vi "Lockin.Sample.vi"(8 "error in (no error)":errorcluster, 11 "Lockin.DAQ":refnum<class "Instrument.DAQ.lvclass">) -> (0 "error out":errorcluster, 2 "Results":T1 {"Results (Dictionary)"."value" format="%#_6p"}, 3 "Lockin.DAQ out":refnum<class "Instrument.DAQ.lvclass">)   [LabVIEW 2019, in "Instrument.Lockin.lvlib" / "Instrument.DAQ.lvclass"]
uses:
  Instrument.DAQ.lvclass
  Typedefs/Results--Cluster.ctl
  Instrument.DAQ.lvclass/Instrument.DAQ.ctl
  <vilib>/Analysis/baseanly.llb/Mean (DBL).vi
  <vilib>/Analysis/NI_AALBase.lvlib
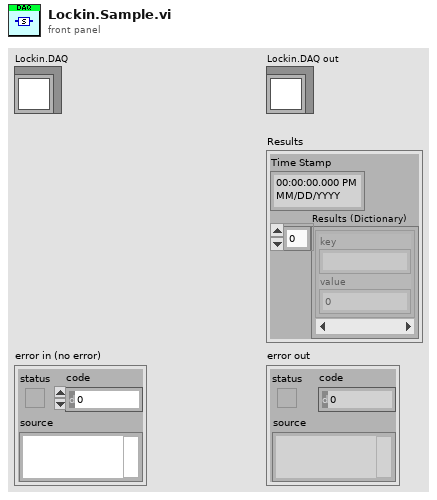
[diagram p1: front panel]
types:
  T1 = typedef "Instrument.Lockin.lvlib/Instrument.DAQ.lvclass/Results--Cluster.ctl" = cluster{"Time Stamp":timestamp, "Results (Dictionary)":cluster{"key":string, "value":dbl}[]}
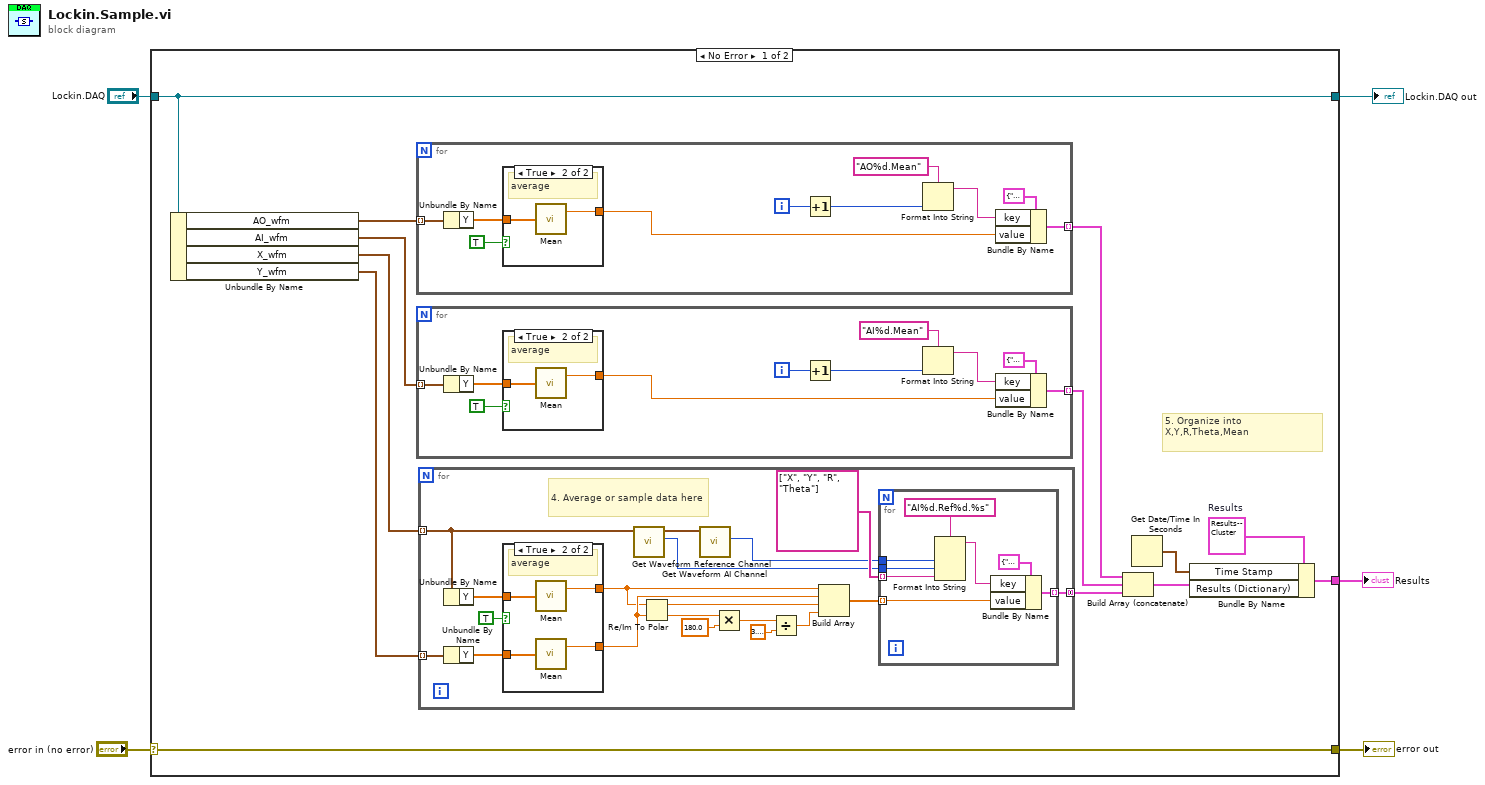
[diagram p0: block diagram]
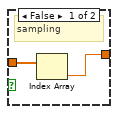
[diagram p2: hidden frame]
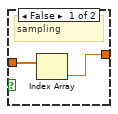
[diagram p3: hidden frame]
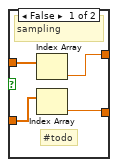
[diagram p4: hidden frame]
diagram:
  n1 = case shown="No Error" "error in (no error)" {
    selector: "error in (no error)" -> [w8 w82]
    tunnel: [w14 _] -> w5
    tunnel: [w8 w82] -> w3
    tunnel: [w7 w83] -> w2
    tunnel: "Lockin.DAQ" -> [w7 w83]
    frame No Error {
      w13 = T1 {"Time Stamp"=timestamp(0 s since 1904-01-01), "Results (Dictionary)"=[]}  # Results
      # "5. Organize into X,Y,R,Theta,Mean"
      n2 = Unbundle By Name(w7) -> ("AO_wfm"=w6:waveform(dbl)[], "AI_wfm"=w11:waveform(dbl)[], "X_wfm"=w10:waveform(dbl)[], "Y_wfm"=w9:waveform(dbl)[])
      n3 = for {
        tunnel: w6 -> [w28] mode=indexing
        tunnel: [w24] -> w12 mode=indexing
        i -> [w23]
        n4 = Unbundle By Name(w28) -> ("Y"=w20:dbl[])
        n5 = case shown="True" TRUE {
          tunnel: w20 -> [w30 w32]
          tunnel: [w29 w31] -> w19
          frame False {
            # "sampling"
            n6 = Index Array(array=w30) -> (element=w29:dbl)  [unwired: 1 in]
          }
          frame True {
            # "average"
            n7 = call-poly <vilib>:"Mean.vi"("X"=w32) -> ("mean"=w31:dbl)  [unwired: 1 out]
          }
        }
        n8 = Increment(x=w23) -> (x+1=w22:i32)
        n9 = Format Into String(format string="AO%d.Mean", w22) -> (resulting string=w26:string)  [unwired: 2 in, 1 out]
        n10 = Bundle By Name(cluster=cluster{"key":string, "value":dbl} {"key"="", "value"=0.0} ("key-value"), "key"=w26, "value"=w19) -> (w24:cluster{"key":string, "value":dbl})
      }
      n11 = for {
        tunnel: w11 -> [w42] mode=indexing
        tunnel: [w38] -> w16 mode=indexing
        i -> [w37]
        n12 = Unbundle By Name(w42) -> ("Y"=w34:dbl[])
        n13 = case shown="True" TRUE {
          tunnel: w34 -> [w44 w46]
          tunnel: [w43 w45] -> w33
          frame False {
            # "sampling"
            n14 = Index Array(array=w44) -> (element=w43:dbl)  [unwired: 1 in]
          }
          frame True {
            # "average"
            n15 = call-poly <vilib>:"Mean.vi"("X"=w46) -> ("mean"=w45:dbl)  [unwired: 1 out]
          }
        }
        n16 = Increment(x=w37) -> (x+1=w36:i32)
        n17 = Format Into String(format string="AI%d.Mean", w36) -> (resulting string=w40:string)  [unwired: 2 in, 1 out]
        n18 = Bundle By Name(cluster=cluster{"key":string, "value":dbl} {"key"="", "value"=0.0} ("key-value"), "key"=w40, "value"=w33) -> (w38:cluster{"key":string, "value":dbl})
      }
      n19 = for {
        tunnel: w10 -> [w49] mode=indexing
        tunnel: w9 -> [w53] mode=indexing
        tunnel: [w55] -> w15 mode=concatenating
        # "4. Average or sample data here"
        n20 = Unbundle By Name(w49) -> ("Y"=w59:dbl[])
        n21 = Unbundle By Name(w53) -> ("Y"=w58:dbl[])
        n22 = case shown="True" TRUE {
          tunnel: w59 -> [w69 w73]
          tunnel: w58 -> [w68 w72]
          tunnel: [w67 w71] -> w57
          tunnel: [w66 w70] -> w56
          frame False {
            # "#todo"
            # "sampling"
            n23 = Index Array(array=w69) -> (element=w66:dbl)  [unwired: 1 in]
            n24 = Index Array(array=w68) -> (element=w67:dbl)  [unwired: 1 in]
          }
          frame True {
            # "average"
            n25 = call-poly <vilib>:"Mean.vi"("X"=w73) -> ("mean"=w70:dbl)  [unwired: 1 out]
            n26 = call-poly <vilib>:"Mean.vi"("X"=w72) -> ("mean"=w71:dbl)  [unwired: 1 out]
          }
        }
        n27 = call "Get Waveform Reference Channel.vi"("Reference in"=w49) -> ("Reference Channel"=w48:i32, "Reference out"=w50:waveform(dbl))  [unwired: 8 in, 1 out]
        n28 = Re/Im To Polar(2:w57, 3:w56) -> (0:w62:dbl, 1:w60:dbl)
        n29 = call "Get Waveform AI Channel.vi"("Reference in"=w50) -> ("AI Channel"=w47:i32)  [unwired: 8 in, 2 out]
        n30 = Multiply(x=w62, y=180.0) -> (x*y=w61:dbl)
        n31 = Divide(x=w61, y=3.141592653589793) -> (x/y=w65:dbl)
        n32 = Build Array(w56, w57, w60, w65) -> (w54:dbl[])
        n33 = for {
          tunnel: w54 -> [w81] mode=indexing
          tunnel: string[] ["X", "Y", "R", "Theta"] -> [w75] mode=indexing
          tunnel: [w79] -> w55 mode=indexing
          tunnel: w48 -> [w76]
          tunnel: w47 -> [w78]
          n34 = Format Into String(format string="AI%d.Ref%d.%s", w78, w76, w75) -> (resulting string=w74:string)  [unwired: 2 in, 1 out]
          n35 = Bundle By Name(cluster=cluster{"key":string, "value":dbl} {"key"="", "value"=0.0} ("key-value"), "key"=w74, "value"=w81) -> (w79:cluster{"key":string, "value":dbl})
        }
      }
      n36 = Build Array (concatenate)(w12, w16, w15) -> (w17:cluster{"key":string, "value":dbl}[])
      n37 = Get Date/Time In Seconds() -> (seconds since 1Jan1904=w18:timestamp)
      n38 = Bundle By Name(cluster=w13, "Time Stamp"=w18, "Results (Dictionary)"=w17) -> (w14:T1)
    }
    frame Error {
    }
  }
  "Results" <- w5
  "error out" <- w3
  "Lockin.DAQ out" <- w2
